vi "OpenCV-FaceDetect.vi"() -> ()   [LabVIEW 2017]
uses:
  IMAQCV/IMAQCV.lvlib
panel:
  in  "type":enum16{"GRAY", "COLOR"}(ring)=enum."COLOR"
  in  "Image Size":T1(ring)
  in  "stop":bool
  out "picture":picture
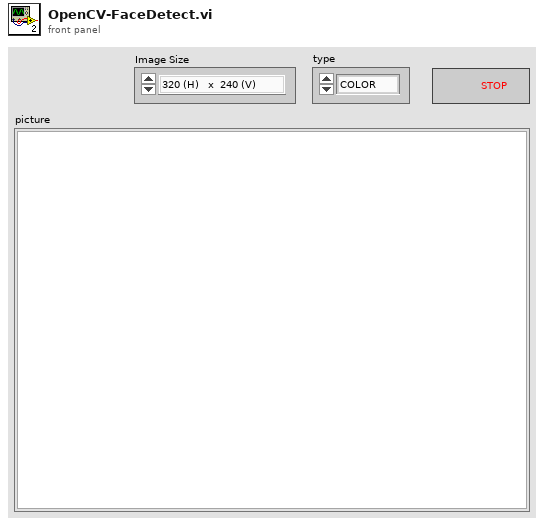
[diagram p1: front panel]
types:
  T1 = enum16{"320 (H)   x  240 (V)", "352(H)    x  288 (V)", "640 (H)   x  480 (V) ", "800 (H)   x  600 (V)", "1024 (H) x  768 (V)", "1280 (H) x  720 (V)", "1280 (H) x  960 (V)", "1280 (H) x 1024 (V)", "1920 (H) x 1080 (V)"}
  T2 = typedef "IMAQCV.lvlib/IMAQCV Image.ctl" = refnum<vi>
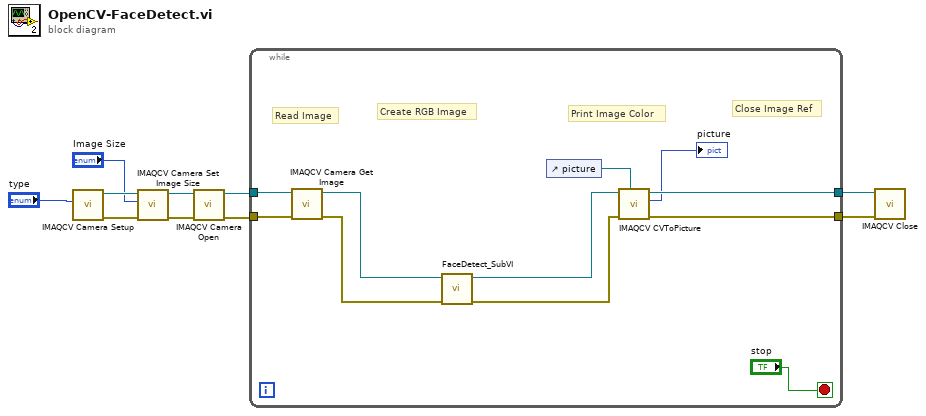
[diagram p0: block diagram]
diagram:
  n1 = call "IMAQCV Camera Setup.vi"("type"="type") -> ("error out"=w6:errorcluster, "image out"=w5:T2)  [unwired: 9 in]
  n2 = call "IMAQCV Camera Set Image Size.vi"("error in (no error)"=w6, "Image Size"="Image Size", "image in"=w5) -> ("error out"=w7:errorcluster, "image out"=w4:T2)  [unwired: 7 in]
  n3 = call "IMAQCV Camera Open.vi"("error in (no error)"=w7, "image in"=w4) -> ("error out"=w8:errorcluster, "image out"=w3:T2)  [unwired: 8 in]
  n4 = while {
    tunnel: w3 -> [w20]
    tunnel: [w18] -> w9
    tunnel: w8 -> [w21]
    tunnel: [w19] -> w10
    stop <- "stop" stop-if-true
    # "Print Image Color"
    # "Close Image Ref"
    # "Create RGB Image"
    # "Read Image"
    n5 = call "IMAQCV Camera Get Image.vi"("error in (no error)"=w21, "image in"=w20) -> ("error out"=w13:errorcluster, "image out"=w12:T2)  [unwired: 8 in]
    n6 = call "FaceDetect_SubVI.vi"("error in (no error)"=w13, "image"=w12) -> ("error out"=w16:errorcluster, "image out"=w15:T2)  [unwired: 8 in]
    n7 = control-ref of="picture"() -> (w11:refnum<vi>)
    n8 = call "IMAQCV CVToPicture.vi"("picture ref"=w11, "error in (no error)"=w16, "image"=w15) -> ("error out"=w19:errorcluster, "picture"=→"picture":picture, "image out"=w18:T2)  [unwired: 6 in]
  }
  n9 = call "IMAQCV Close.vi"("error in (no error)"=w10, "Image"=w9) -> ()  [unwired: 9 in, 1 out]
